vi "GE 5565PIORC.DMA.Scatter-Gather.Link Block Descriptors.vi"(9 "error in (no error)":errorcluster, 11 "Block Descriptors":T1[](array[typedef]) {"descriptor params"."data ptr (lower)" format="%.0x"; "descriptor params"."data ptr (upper)" format="%.0x"; "descriptor params"."data size" format="%.0x"; "descriptor params"."next descriptor ptr" format="%.0x"; "descriptor size" format="%08x"; "descriptor ptr (RFM)" format="%08x"; "descriptor ptr (VISA)" format="%08x"}) -> (1 "error out":errorcluster, 3 "Linked Block Descriptors":T1[](array[typedef]) {"descriptor params"."data ptr (lower)" format="%.0x"; "descriptor params"."data ptr (upper)" format="%.0x"; "descriptor params"."data size" format="%.0x"; "descriptor params"."next descriptor ptr" format="%.0x"; "descriptor size" format="%08x"; "descriptor ptr (RFM)" format="%08x"; "descriptor ptr (VISA)" format="%08x"})   [LabVIEW 2016, in "GE 5565PIORC.lvclass"]
doc: "Modifies the pointers for each Block Descriptor in the <B>Block Descriptors</B> array to ensure that each element points to the location of the next descriptor in memory."
uses:
  GE 5565PIORC.lvclass
  Typedefs/GE 5565PIORC.Typedef.DMA Block Descriptor.ctl
  Typedefs/GE 5565PIORC.Typedef.DMA Block Descriptor Params.ctl
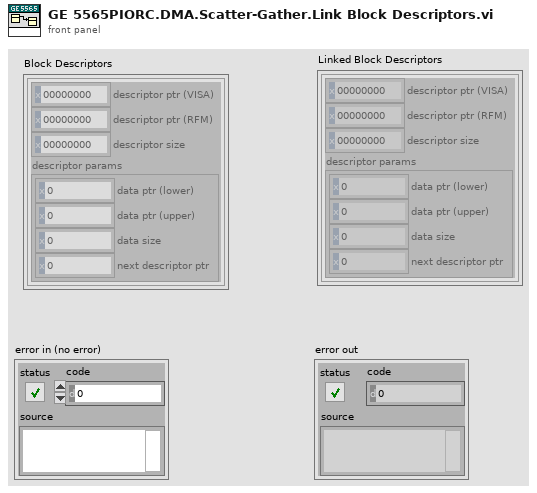
[diagram p1: front panel]
types:
  T1 = typedef "GE 5565PIORC.lvclass/GE 5565PIORC.Typedef.DMA Block Descriptor.ctl" = cluster{"descriptor ptr (VISA)":u32, "descriptor ptr (RFM)":u32, "descriptor size":u32, "descriptor params":T2}
  T2 = typedef "GE 5565PIORC.lvclass/GE 5565PIORC.Typedef.DMA Block Descriptor Params.ctl" = cluster{"data ptr (lower)":u32, "data ptr (upper)":u32, "data size":u32, "next descriptor ptr":u32}
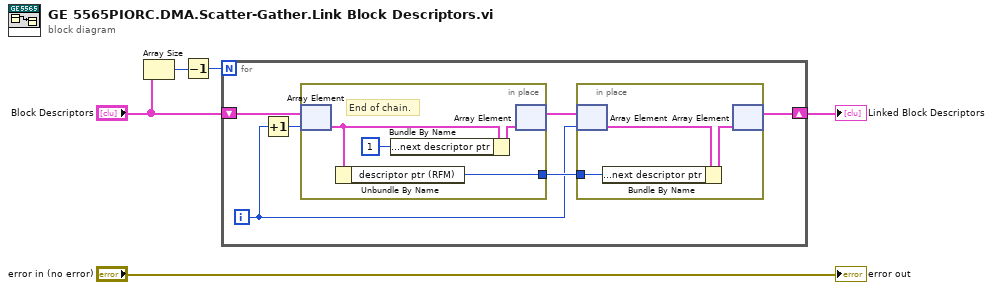
[diagram p0: block diagram]
diagram:
  n1 = Array Size(array="Block Descriptors") -> (size(s)=w4:i32)
  n2 = Decrement(x=w4) -> (x-1=w3:i32)
  n3 = for {
    N: w3 -> [_]
    shift-right: [w8] -> w1
    shift-left: "Block Descriptors" -> [w10]
    i -> [w6]
    n4 = Increment(x=w6) -> (x+1=w11:i32)
    n5 = in-place {
      in-place-border: [w12] -> w7
      # "End of chain."
      n6 = in-place-array #1(w10, w11) -> (w15:T1)
      n7 = Unbundle By Name(w15) -> ("descriptor ptr (RFM)"=w12:u32)
      n8 = Bundle By Name(cluster=w15, "descriptor params.next descriptor ptr"=u32 1 ("next descriptor ptr")) -> (w14:T1)
      n9 = in-place-array #1(w14) -> (w9:T1[])  [unwired: 1 out]
    }
    n10 = in-place {
      in-place-border: w7 -> [w16]
      n11 = in-place-array #2(w9, w6) -> (w18:T1)
      n12 = Bundle By Name(cluster=w18, "descriptor params.next descriptor ptr"=w16) -> (w17:T1)
      n13 = in-place-array #2(w17) -> (w8:T1[])  [unwired: 1 out]
    }
  }
  "Linked Block Descriptors" <- w1
  "error out" <- "error in (no error)"
